vi "DAQmx Create Channel (DI-Digital Input).vi"(0 "task in":refnum<k21>, 5 "lines":tag, 7 "name to assign":string, 9 "line grouping":i32(ring)=1 items=["one channel for each line", "one channel for all lines"], 11 "error in":errorcluster) -> (4 "task out":refnum<k21>, 15 "error out":errorcluster)   [LabVIEW 2011]
doc: "Creates channel(s) to measure digital signals. You can group digital lines into one digital channel or separate them into multiple digital channels. If you specify one or more entire ports in the <B>lines</B> input by using port physical channel names, you cannot separate the ports into multiple channels. To separate ports into multiple channels, use this VI multiple times with a different port each time."
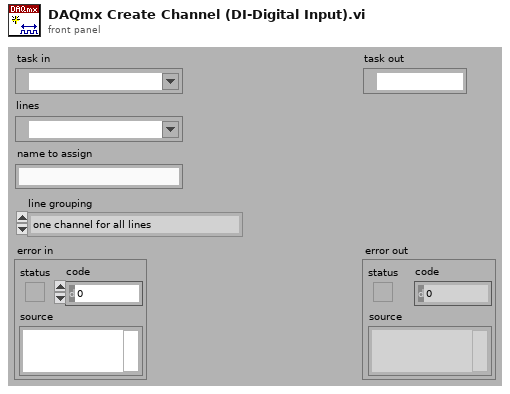
[diagram p1: front panel]
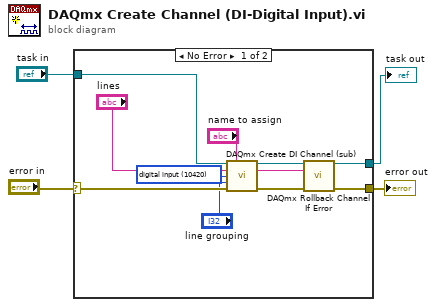
[diagram p0: block diagram]
diagram:
  n1 = case shown="No Error" "error in" {
    selector: "error in" -> [w13 w17]
    tunnel: [w8 w17] -> w4
    tunnel: "task in" -> [w14 w16]
    tunnel: [w5 w16] -> w1
    frame No Error {
      w11 = 10420 items=["digital input"=10420] ("measurement type")
      n2 = call "DAQmx Create DI Channel (sub).vi"("task in"=w14, "virtual channel name"="name to assign", "physical channel name"="lines", "measurement type"=w11, "line grouping"="line grouping", "error in"=w13) -> ("task out"=w7:refnum<k21>, "channel names"=w6:string, "error out"=w9:errorcluster)  [unwired: 7 out]
      n3 = call "DAQmx Rollback Channel If Error.vi"("task in"=w7, "channel names"=w6, "error in"=w9) -> ("task out"=w5:refnum<k21>, "error out"=w8:errorcluster)  [unwired: 11 out]
    }
    frame Error {
    }
  }
  "error out" <- w4
  "task out" <- w1
